vi "Calculate Distance.vi"(10 "Y Resolution":i32, 11 "Target Height (px)":dbl) -> (2 "real size to pixle ration (in/px)":dbl, 3 "Distance (in)":dbl)   [LabVIEW 2012]
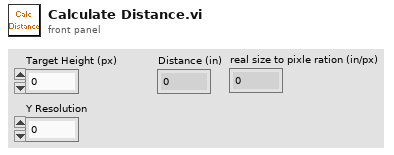
[diagram p1: front panel]
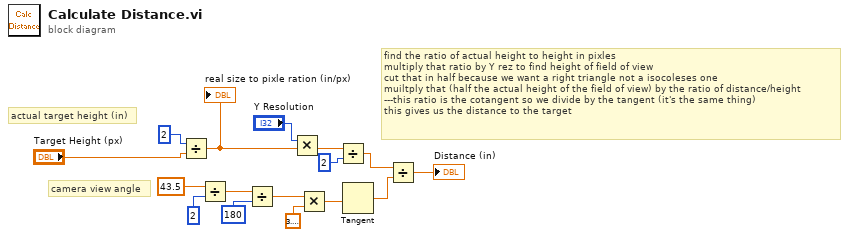
[diagram p0: block diagram]
diagram:
  # "find the ratio of actual height to height in pixles\nmultiply that ratio by Y rez to find height of field of view\ncut that in half because we want a right triangle not a isocoleses one\nmuiltply that (half the actual height of the field of view) by the ratio of distance/height\n---this ratio is the cotangent so we divide by the tangent (it's the same thing)\nthis gives us the distance to the target"
  # "camera view angle"
  # "actual target height (in)"
  n1 = Divide(x=2, y="Target Height (px)") -> (x/y=w12:dbl)
  "real size to pixle ration (in/px)" <- w12
  n2 = Divide(x=43.5, y=2) -> (x/y=w6:dbl)
  n3 = Divide(x=w6, y=180) -> (x/y=w7:dbl)
  n4 = Multiply(x="Y Resolution", y=w12) -> (x*y=w13:dbl)
  n5 = Multiply(x=w7, y=3.141592653589793) -> (x*y=w5:dbl)
  n6 = Divide(x=w13, y=2) -> (x/y=w15:dbl)
  n7 = Tangent(1:w5) -> (0:w16:dbl)
  n8 = Divide(x=w15, y=w16) -> (x/y=→"Distance (in)":dbl)
